vi "ORTForceCurves.vi"() -> ()   [LabVIEW 2016]
uses:
  controls/ORTForceCurveEnumTypeDef.ctl
  controls/Enum.ctl
  <vilib>/rvi/errors/niLvFpgaAdjustHostInterfaceError.vi
  <vilib>/Utility/error.llb/Error Cluster From Error Code.vi
  <vilib>/RVI Host/nirviSupport.llb/nirviErrorClusterFromErrorCode.vi
  controls/FPGAVIreferenceTypeDef.ctl
  <vilib>/rvi/interface/nirviReadWriteControl/nirviReadWriteControl.xnode
  FPGA Bitfiles/qnmController797_usbRIO_controllerFPGAmu.lvbitx
  <vilib>/rvi/interface/nirviMethod/nirviMethod.xnode
  <vilib>/rvi/errors/niLvFpgaMergeErrorWithErrorCode.vi
  NiFpgaLv.dll
  <vilib>/FPGAPlugInAG/USB-7856R OEM/niLvFpga_ReadFifo_USB-7856R OEM.vi
  <vilib>/rvi/interface/nirviMethod/StockFPGA_InlinedMethodWaitForSingleIRQ.vi
  <vilib>/FPGAPlugInAG/USB-7856R OEM/niLvFpga_WaitOnIrq_USB-7856R OEM.vi
  <vilib>/FPGAPlugInAG/USB-7856R OEM/niLvFpga_AcknowledgeIrq_USB-7856R OEM.vi
panel:
  in  "Refresh":i32=100 format="%.0fms"
  in  "Raw":bool
  in  "Plot Force Distance":bool=TRUE
  out "Time Domain":waveform(dbl)(graph)
  out "Force Distance":cluster{dbl[], "Data":dbl[]}(graph)
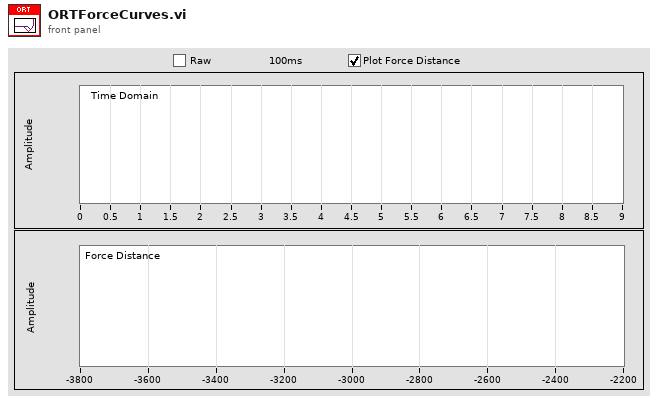
[diagram p1: front panel]
types:
  T1 = typedef "ORTForceCurveEnumTypeDef.ctl" = enum16{"Init", "AskForNewCurve", "Update.CalibZ", "Refresh.Graph", "WaitForEvents", "Close"}
  T2 = typedef "Enum.ctl" = enum16{"Init", "Read", "Write"}
  T3 = enum32{"Bad", "Idle", "Run top level", "Running"}
  T4 = typedef "FPGAVIreferenceTypeDef.ctl" = refnum<k20>
  T5 = cluster{"hdt.int.s.transferSource":u8, "hdt.int.p.useInternalMemStartPos":bool, "hdt.int.p.memStartPos":fxp<+,14,14>, "hdt.int.p.readLength":u16, "hdt.int.p.readFwd":bool, "hdt.int.p.memReadDec":u16, "hdt.int.p.startTransfer":bool}
  T6 = cluster{"inputSensitivity":dbl, "outputSensitivity":dbl}
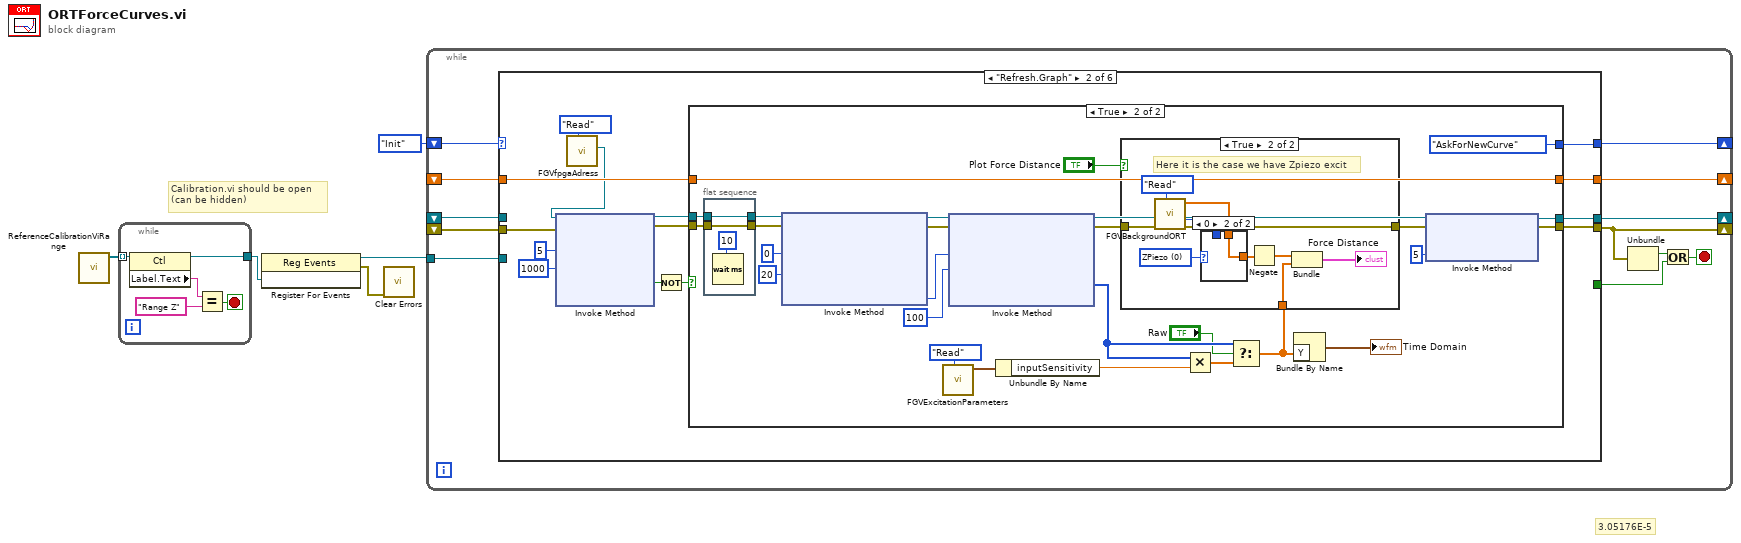
[diagram p0: block diagram]
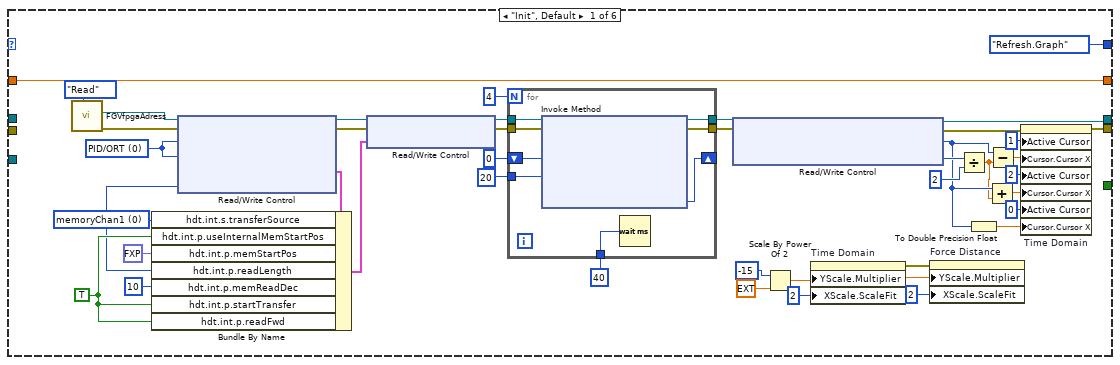
[diagram p2: hidden frame]
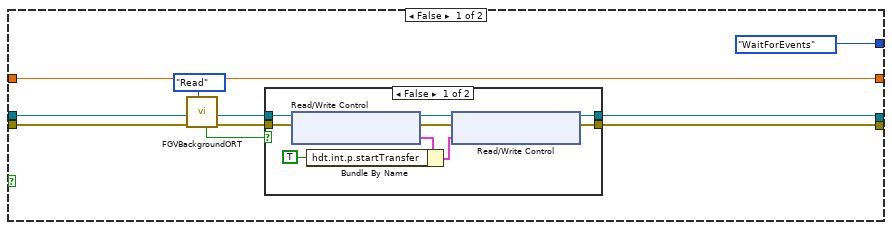
[diagram p3: hidden frame]
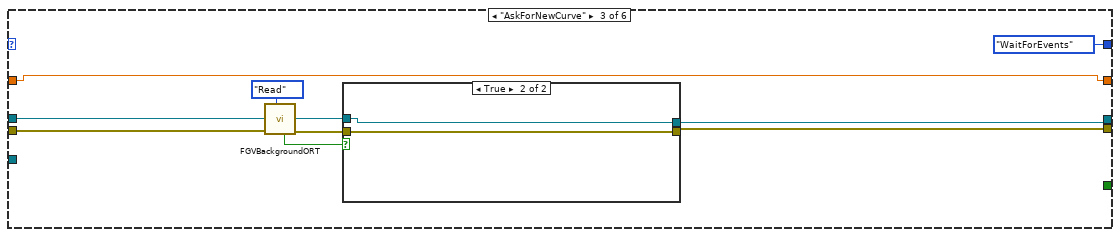
[diagram p7: hidden frame]
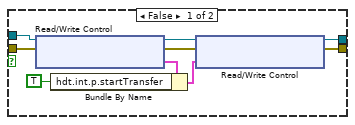
[diagram p8: hidden frame]
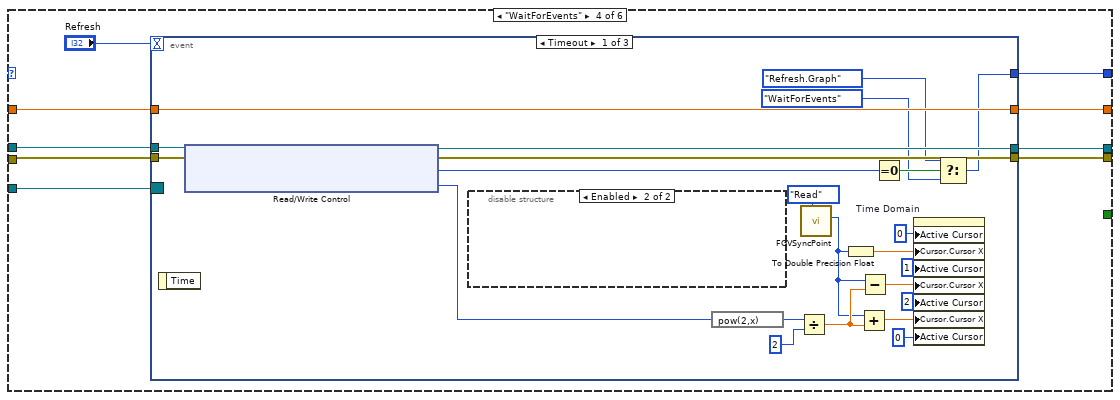
[diagram p9: hidden frame]
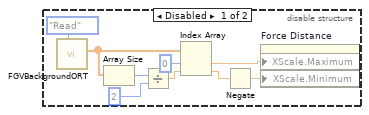
[diagram p10: hidden frame]
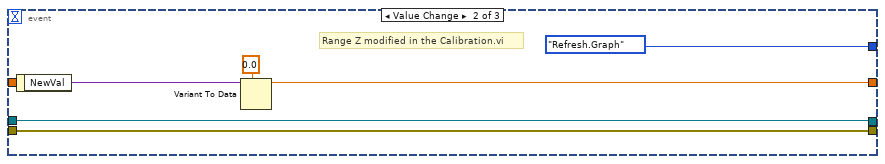
[diagram p11: hidden frame]
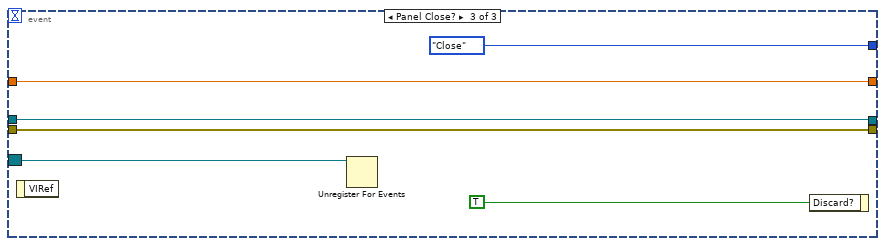
[diagram p12: hidden frame]
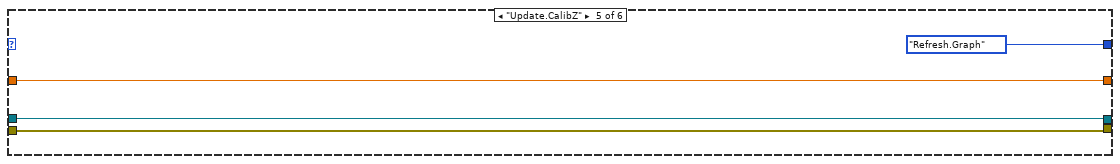
[diagram p13: hidden frame]
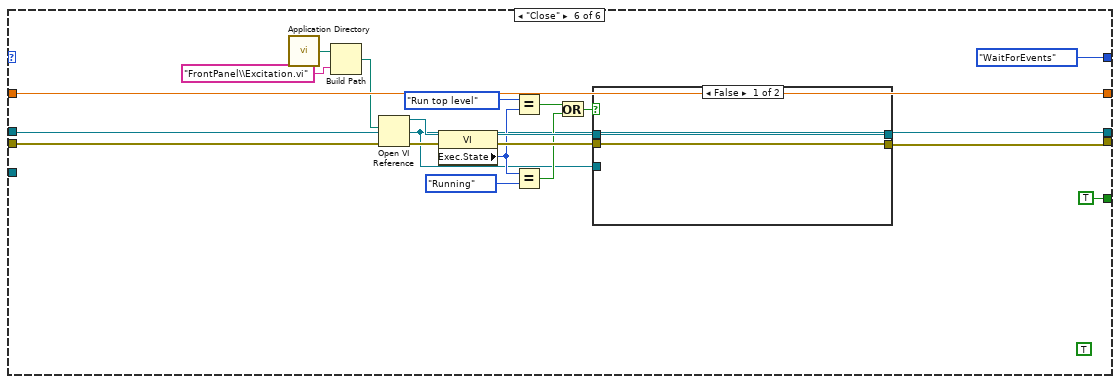
[diagram p14: hidden frame]
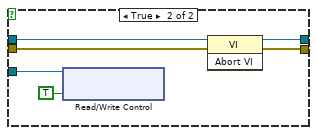
[diagram p15: hidden frame]
diagram:
  # "3.05176E-5"
  # "Calibration.vi should be open\n(can be hidden)"
  n1 = call "ReferenceCalibrationViRange.vi"() -> ("Ranges"=w5:refnum<vi>[])  [unwired: 8 in, 3 out]
  n2 = while {
    tunnel: w5 -> [w10] mode=indexing
    tunnel: [w7] -> w4
    stop <- w6 stop-if-true
    n3 = property class="Ctl"(reference=w10) -> (reference out=w7:refnum<vi>, "Label.Text"=w9:string)  [unwired: 1 in, 1 out]
    n4 = Equal?(x=w9, y="Range Z") -> (x = y?=w6:bool)
  }
  n5 = register-events(w4) -> (reference out=w3:refnum<event-registration>, error out=w1:errorcluster)  [unwired: 2 in]
  n6 = call <vilib>:"Clear Errors.vi"("error in (no error)"=w1) -> ()  [unwired: 5 in, 2 out]
  n7 = while {
    shift-right: [w21] -> _
    shift-left: _ -> [w20]
    shift-right: [w19] -> _
    shift-left: ORTForceCurveEnumTypeDef."Init" -> [w22]
    tunnel: w3 -> [w18]
    shift-right: [w17] -> _
    shift-left: _ -> [w16]
    shift-right: [w14] -> _
    shift-left: _ -> [w15]
    stop <- w11 stop-if-true
    n8 = case shown="\"Refresh.Graph\"" w22 {
      tunnel: [w56 w81 w151 w172 w226 w227] -> w21
      tunnel: w20 -> [_ _ w152 w173 w226 w227]
      tunnel: [ORTForceCurveEnumTypeDef."Refresh.Graph" w80 ORTForceCurveEnumTypeDef."WaitForEvents" w176 ORTForceCurveEnumTypeDef."Refresh.Graph" ORTForceCurveEnumTypeDef."WaitForEvents"] -> w19
      tunnel: [_ _ _ _ _ TRUE ("Discard?")] -> w12
      tunnel: w18 -> [_ _ _ w177 _ _]
      tunnel: [w60 w78 w153 w175 w224 w242] -> w17
      tunnel: w16 -> [w60 w79 w153 w174 w224 w242]
      tunnel: [w57 w76 w150 w170 w223 w228] -> w14
      tunnel: w15 -> [_ w77 w155 w171 w223 w245]
      frame "Init", Default {
        w23 = u8 0 items=["PID/ORT", "SICM"] ("hdt.mainOutStreamSelect")
        w48 = TRUE ("hdt.int.p.startTransfer")
        w45 = u8 0 items=["memoryChan1", "memoryChan2", "processVarFixedNoPts", "processVarStream"] ("hdt.int.s.transferSource")
        n9 = call "FGVfpgaAdress.vi"("Enum"=Enum."Read") -> ("error out"=w43:errorcluster, "FPGA VI Reference Out"=w42:T4)  [unwired: 5 in, 4 out]
        n10 = xnode "Read/Write Control"("FPGA VI Reference In"=w42, "error in"=w43, "hdt.mainOutStreamSelect"=w23, "hdt.int.p.memWriteSource"=w23) -> ("FPGA VI Reference Out"=w40:T4, "error out"=w37:errorcluster, "hdt.int.p.readParams"=w44:T5, "ort.p.waveSize"=w41:u16)
        n11 = Bundle By Name(cluster=w44, "hdt.int.s.transferSource"=w45, "hdt.int.p.useInternalMemStartPos"=w48, "hdt.int.p.memStartPos"=fxp<+,14,14> 0.0, "hdt.int.p.readLength"=w41, "hdt.int.p.memReadDec"=u16 10, "hdt.int.p.startTransfer"=w48, "hdt.int.p.readFwd"=w48) -> (w36:T5)
        n12 = xnode "Read/Write Control"("FPGA VI Reference In"=w40, "error in"=w37, "hdt.int.p.readParams"=w36) -> ("FPGA VI Reference Out"=w39:T4, "error out"=w38:errorcluster)
        n13 = for {
          N: 4 -> [_]
          shift-right: [w69] -> _
          shift-left: u32 0 ("Elements Remaining") -> [w70]
          tunnel: w39 -> [w68]
          tunnel: [w66] -> w50
          tunnel: 20 ("Timeout (ms)") -> [w67]
          tunnel: u32 40 ("milliseconds to wait") -> [w65]
          tunnel: w38 -> [w72]
          tunnel: [w71] -> w49
          n14 = xnode "Invoke Method"("FPGA VI Reference In"=w68, "error in"=w72, "Number of Elements"=w70, "Timeout (ms)"=w67) -> ("FPGA VI Reference Out"=w66:T4, "error out"=w71:errorcluster, "Elements Remaining"=w69:u32)  [unwired: 1 out]
          n15 = Wait (ms)(milliseconds to wait=w65) -> ()  [unwired: 1 out]
        }
        n16 = xnode "Read/Write Control"("FPGA VI Reference In"=w50, "error in"=w49) -> ("FPGA VI Reference Out"=w56:T4, "error out"=w51:errorcluster, "ort.p.methodParams.ort.p.syncPoint"=w27:u16, "ort.p.methodParams.ort.p.winSizeP2"=w31:u16)
        n17 = Scale By Power Of 2(n=i16 -15, x=ext 1.0) -> (x*2^n=w52:ext)
        n18 = property on="Time Domain" class="WFGraph (strict)"("YScale.Multiplier"=w52, "XScale.ScaleFit"=u8 2 ("X Scale.Scale Fit")) -> (error out=w55:errorcluster)  [unwired: 2 in, 1 out]
        n19 = property on="Force Distance" class="XYGraph (strict)"(error in=w55, "YScale.Multiplier"=w52, "XScale.ScaleFit"=u8 2 ("X Scale.Scale Fit")) -> ()  [unwired: 1 in, 2 out]
        n20 = Divide(x=w31, y=u16 2) -> (x/y=w26:dbl)
        n21 = To Double Precision Float(number=w27) -> (double precision float=w35:dbl)
        n22 = Add(x=w27, y=w26) -> (x+y=w28:dbl)
        n23 = Subtract(x=w27, y=w26) -> (x-y=w29:dbl)
        n24 = property on="Time Domain" class="WFGraph (strict)"(error in=w51, "Active Cursor"=u32 1, "Cursor.Cursor X"=w29, "Active Cursor"=u32 2, "Cursor.Cursor X"=w28, "Active Cursor"=u32 0, "Cursor.Cursor X"=w35) -> (error out=w57:errorcluster)  [unwired: 1 in, 1 out]
      }
      frame "Refresh.Graph" {
        n25 = call "FGVfpgaAdress.vi"("Enum"=Enum."Read") -> ("FPGA VI Reference Out"=w74:T4)  [unwired: 5 in, 5 out]
        n26 = xnode "Invoke Method"("FPGA VI Reference In"=w74, "error in"=w77, "IRQ Number(s)"=5, "Timeout (ms)"=1000) -> ("FPGA VI Reference Out"=w82:T4, "error out"=w83:errorcluster, "Timed Out"=w85:bool)  [unwired: 1 out]
        n27 = Not(x=w85) -> (.not. x?=w86:bool)
        n28 = case shown="True" w86 {
          tunnel: [w92 w133] -> w81
          tunnel: [w91 w132] -> w76
          tunnel: w82 -> [w93 w109]
          tunnel: w83 -> [w89 w120]
          tunnel: [ORTForceCurveEnumTypeDef."WaitForEvents" ORTForceCurveEnumTypeDef."AskForNewCurve"] -> w80
          tunnel: w79 -> [w94 w115]
          tunnel: [w94 w115] -> w78
          frame False {
            n29 = call "FGVBackgroundORT.vi"("Enum"=Enum."Read", "error in"=w89) -> ("error out"=w88:errorcluster, "Corrected...Out"=w87:bool)  [unwired: 5 in, 3 out]
            n30 = case shown="False" w87 {
              tunnel: w93 -> [w104 w106]
              tunnel: [w103 w106] -> w92
              tunnel: [w102 w105] -> w91
              tunnel: w88 -> [w96 w105]
              frame False {
                n31 = xnode "Read/Write Control"("FPGA VI Reference In"=w104, "error in"=w96) -> ("FPGA VI Reference Out"=w98:T4, "error out"=w97:errorcluster, "hdt.int.p.readParams"=w101:T5)
                n32 = Bundle By Name(cluster=w101, "hdt.int.p.startTransfer"=TRUE) -> (w100:T5)
                n33 = xnode "Read/Write Control"("FPGA VI Reference In"=w98, "error in"=w97, "hdt.int.p.readParams"=w100) -> ("FPGA VI Reference Out"=w103:T4, "error out"=w102:errorcluster)
              }
              frame True {
              }
            }
          }
          frame True {
            n34 = flat-sequence {
              tunnel: [w148] -> w121
              tunnel: w109 -> [w148]
              tunnel: w120 -> [w147]
              tunnel: [w147] -> w108
              frame #0 {
                n35 = Wait (ms)(milliseconds to wait=u32 10) -> ()  [unwired: 1 out]
              }
            }
            n36 = xnode "Invoke Method"("FPGA VI Reference In"=w121, "error in"=w108, "Number of Elements"=u32 0, "Timeout (ms)"=20) -> ("FPGA VI Reference Out"=w125:T4, "error out"=w124:errorcluster, "Elements Remaining"=w128:u32)  [unwired: 1 out]
            n37 = call "FGVExcitationParameters.vi"("Enum"=Enum."Read") -> ("Sensitivities Out"=w113:T6)  [unwired: 6 in, 4 out]
            n38 = xnode "Invoke Method"("FPGA VI Reference In"=w125, "error in"=w124, "Number of Elements"=w128, "Timeout (ms)"=100) -> ("FPGA VI Reference Out"=w111:T4, "error out"=w110:errorcluster, "Data"=w129:i16[])  [unwired: 1 out]
            n39 = Unbundle By Name(w113) -> ("inputSensitivity"=w112:dbl)
            n40 = Multiply(x=w129, y=w112) -> (x*y=w130:dbl[])
            n41 = Select(t=w129, s="Raw", f=w130) -> (s? t:f=w123:dbl[])
            n42 = case shown="True" "Plot Force Distance" {
              tunnel: w123 -> [_ w144]
              tunnel: [w134 w142] -> w118
              tunnel: w110 -> [w134 w141]
              frame False {
              }
              frame True {
                w139 = u16 0 items=["ZPiezo", "Photothermal"] ("Type")
                # "Here it is the case we have Zpiezo excit"
                n43 = call "FGVBackgroundORT.vi"("Enum"=Enum."Read", "error in"=w141) -> ("error out"=w142:errorcluster, "arrayOut"=w138:i16[], "Wave Out Shifted"=w135:dbl[])  [unwired: 5 in, 2 out]
                n44 = case shown="0" w139 {
                  tunnel: [w145 w146] -> w140
                  tunnel: w135 -> [_ w146]
                  tunnel: w138 -> [w145 _]
                  frame 1, Default {
                  }
                  frame 0 {
                  }
                }
                n45 = Negate(x=w140) -> (-x=w136:dbl[])
                n46 = Bundle(w136, "Data"=w144) -> (→"Force Distance":cluster{dbl[], "Data":dbl[]})  [unwired: 1 in]
              }
            }
            n47 = Bundle By Name("Y"=w123) -> (→"Time Domain":waveform(dbl))  [unwired: 1 in]
            n48 = xnode "Invoke Method"("FPGA VI Reference In"=w111, "error in"=w118, "IRQ Number(s)"=5) -> ("FPGA VI Reference Out"=w133:T4, "error out"=w132:errorcluster)
          }
        }
      }
      frame "AskForNewCurve" {
        n49 = call "FGVBackgroundORT.vi"("Enum"=Enum."Read", "error in"=w155) -> ("error out"=w157:errorcluster, "Corrected...Out"=w156:bool)  [unwired: 5 in, 3 out]
        n50 = case shown="True" w156 {
          tunnel: [w167 w168] -> w151
          tunnel: [w166 w169] -> w150
          tunnel: w157 -> [w160 w169]
          tunnel: w152 -> [w159 w168]
          frame False {
            n51 = xnode "Read/Write Control"("FPGA VI Reference In"=w159, "error in"=w160) -> ("FPGA VI Reference Out"=w162:T4, "error out"=w161:errorcluster, "hdt.int.p.readParams"=w165:T5)
            n52 = Bundle By Name(cluster=w165, "hdt.int.p.startTransfer"=TRUE) -> (w164:T5)
            n53 = xnode "Read/Write Control"("FPGA VI Reference In"=w162, "error in"=w161, "hdt.int.p.readParams"=w164) -> ("FPGA VI Reference Out"=w167:T4, "error out"=w166:errorcluster)
          }
          frame True {
          }
        }
      }
      frame "WaitForEvents" {
        n54 = event shown="[0] Timeout" {
          selector: w177 -> [_ _ w219]
          dyn-events: _ -> [_ _ _]
          timeout: "Refresh" -> [_ _ _]
          tunnel: [w195 ORTForceCurveEnumTypeDef."Refresh.Graph" ORTForceCurveEnumTypeDef."Close"] -> w176
          tunnel: [w199 w214 w220] -> w175
          tunnel: w174 -> [w199 _ w220]
          tunnel: w173 -> [w198 w212 w218]
          tunnel: [w200 w212 w218] -> w172
          tunnel: w171 -> [w191 w211 w217]
          tunnel: [w201 w211 w217] -> w170
          event Timeout {
            n55 = event-data() -> ()  [unwired: 1 in, 1 out]
            n56 = xnode "Read/Write Control"("FPGA VI Reference In"=w198, "error in"=w191) -> ("FPGA VI Reference Out"=w200:T4, "error out"=w201:errorcluster, "hdt.int.p.readParams.hdt.int.s.transferSource"=w197:u8, "ort.p.methodParams.ort.p.winSizeP2"=w190:u16)
            n57 = disable-structure shown="Enabled" {
              frame Disabled {
                n58 = call "FGVBackgroundORT.vi"("Enum"=Enum."Read") -> ("Wave Out"=w207:dbl[])  [unwired: 6 in, 4 out]
                n59 = Array Size(array=w207) -> (size(s)=w206:i32)
                n60 = Divide(x=w206, y=2) -> (x/y=w204:dbl)
                n61 = Index Array(array=w207, index #1=0 ("index"), index #2=w204) -> (element #1=w209:dbl, element #2=w203:dbl)
                n62 = Negate(x=w203) -> (-x=w202:dbl)
                n63 = property on="Force Distance" class="XYGraph (strict)"("XScale.Maximum"=w209, "XScale.Minimum"=w202) -> ()  [unwired: 2 in, 2 out]
              }
              frame Enabled {
              }
            }
            n64 = expression code="pow(2,x)"(w190) -> (w183:u16)
            n65 = Divide(x=w183, y=u16 2) -> (x/y=w184:dbl)
            n66 = call "FGVSyncPoint.vi"("Enum"=Enum."Read") -> ("SyncPointOut"=w179:u16)  [unwired: 9 in, 1 out]
            n67 = To Double Precision Float(number=w179) -> (double precision float=w181:dbl)
            n68 = Add(x=w179, y=w184) -> (x+y=w185:dbl)
            n69 = Subtract(x=w179, y=w184) -> (x-y=w186:dbl)
            n70 = Equal To 0?(x=w197) -> (x = 0?=w196:bool)
            n71 = property on="Time Domain" class="WFGraph (strict)"("Active Cursor"=u32 0, "Cursor.Cursor X"=w181, "Active Cursor"=u32 1, "Cursor.Cursor X"=w186, "Active Cursor"=u32 2, "Cursor.Cursor X"=w185, "Active Cursor"=u32 0) -> ()  [unwired: 2 in, 2 out]
            n72 = Select(t=ORTForceCurveEnumTypeDef."Refresh.Graph", s=w196, f=ORTForceCurveEnumTypeDef."WaitForEvents") -> (s? t:f=w195:T1)
          }
          event Value Change {
            # "Range Z modified in the Calibration.vi"
            n73 = event-data() -> ("NewVal"=w216:variant)  [unwired: 1 in]
            n74 = Variant To Data(type=0.0, Variant=w216) -> (data=w214:dbl)  [unwired: 1 in, 1 out]
          }
          event Panel Close? {
            n75 = event-data() -> ()  [unwired: 1 in, 1 out]
            n76 = Unregister For Events(event registration refnum=w219) -> ()  [unwired: 1 in, 1 out]
            n77 = event-data("Discard?"=TRUE) -> ()  [unwired: 1 in, 1 out]
          }
        }
      }
      frame "Update.CalibZ" {
      }
      frame "Close" {
        (unwired) TRUE
        n78 = call <vilib>:"Application Directory.vi"() -> ("Application Directory"=w240:path)
        n79 = Build Path(base path=w240, name or relative path="FrontPanel\\Excitation.vi") -> (appended path=w239:path)
        n80 = Open VI Reference(vi path=w239, error in (no error)=w245) -> (vi reference=w229:refnum<vi>, error out=w230:errorcluster)  [unwired: 4 in]
        n81 = property class="VI"(reference=w229, error in=w230) -> (reference out=w238:refnum<vi>, error out=w237:errorcluster, "Exec.State"=w232:T3)
        n82 = Equal?(x=T3."Run top level" ("Execution:State"), y=w232) -> (x = y?=w234:bool)
        n83 = Equal?(x=w232, y=T3."Running" ("Execution:State")) -> (x = y?=w233:bool)
        n84 = Or(x=w234, y=w233) -> (x .or. y?=w231:bool)
        n85 = case shown="False" w231 {
          tunnel: [w246 w250] -> w228
          tunnel: [w247 w252] -> _
          tunnel: w238 -> [w247 w253]
          tunnel: w237 -> [w246 w251]
          tunnel: w227 -> [_ w249]
          frame False {
          }
          frame True {
            n86 = xnode "Read/Write Control"("FPGA VI Reference In"=w249, "aio.o.disableExc"=TRUE) -> ()  [unwired: 1 in, 2 out]
            n87 = invoke class="VI" method="Abort VI"(reference=w253, error in=w251) -> (reference out=w252:refnum<vi>, error out=w250:errorcluster)  [unwired: 1 in, 1 out]
          }
        }
      }
    }
    n88 = Unbundle(w14) -> ("status"=w13:bool)  [unwired: 2 out]
    n89 = Or(x=w13, y=w12) -> (x .or. y?=w11:bool)
  }
